vi "serial_com_port.vi"() -> ()   [LabVIEW 2024]
uses:
  <vilib>/Instr/_visa.llb/VISA Configure Serial Port (Instr).vi
panel:
  out "fail message":string
  out "error out 4":errorcluster
  out "error out 3":errorcluster
  out "x+y":dbl
  in  "y":dbl
  in  "x":dbl
  out "pass message":string
  out "error out 2":errorcluster
  in  "COM Port 2":refnum<visa-resource-name>
  out "error out":errorcluster
  in  "COM Port 1":refnum<visa-resource-name>
  in  "stop":bool
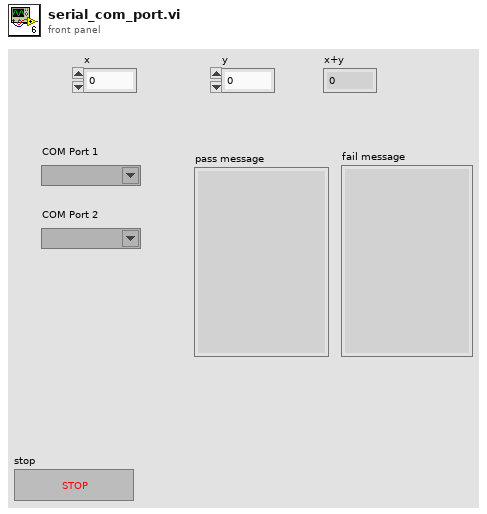
[diagram p1: front panel]
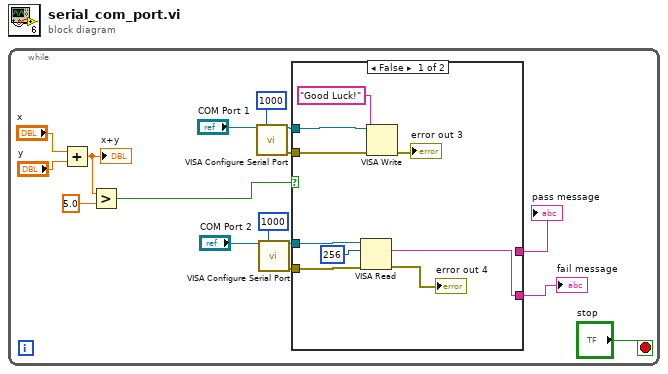
[diagram p0: block diagram]
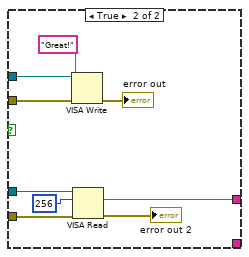
[diagram p2: hidden frame]
diagram:
  n1 = while {
    stop <- "stop" stop-if-true
    n2 = Add(x="x", y="y") -> (x+y=w4:dbl)
    "x+y" <- w4
    n3 = Greater?(x=w4, y=5.0) -> (0:w1:bool)
    n4 = call-poly "VISA Configure Serial Port"("VISA resource name"="COM Port 1", "timeout (10sec)"=u32 1000) -> ("VISA resource name out"=w14:refnum<visa-resource-name>, "error out"=w13:errorcluster)  [unwired: 12 in]
    n5 = call-poly "VISA Configure Serial Port"("VISA resource name"="COM Port 2", "timeout (10sec)"=u32 1000) -> ("VISA resource name out"=w11:refnum<visa-resource-name>, "error out"=w10:errorcluster)  [unwired: 12 in]
    n6 = case shown="False" w1 {
      tunnel: w14 -> [w21 w34]
      tunnel: w13 -> [w20 w32]
      tunnel: w11 -> [w19 w30]
      tunnel: w10 -> [w18 w29]
      tunnel: [_ w26] -> w9
      tunnel: [w17 _] -> w2
      frame False {
        n7 = VISA Read(VISA resource name=w19, byte count=u32 256, error in (no error)=w18) -> (read buffer=w17:string, error out=→"error out 4":errorcluster)  [unwired: 2 out]
        n8 = VISA Write(VISA resource name=w21, write buffer="Good Luck!", error in (no error)=w20) -> (error out=→"error out 3":errorcluster)  [unwired: 2 out]
      }
      frame True {
        n9 = VISA Write(VISA resource name=w34, write buffer="Great!", error in (no error)=w32) -> (error out=→"error out":errorcluster)  [unwired: 2 out]
        n10 = VISA Read(VISA resource name=w30, byte count=u32 256, error in (no error)=w29) -> (read buffer=w26:string, error out=→"error out 2":errorcluster)  [unwired: 2 out]
      }
    }
    "pass message" <- w9
    "fail message" <- w2
  }
